vi "FFT1D_LabVIEW.vi"(7 "Iteration":i32, 11 "Samples":i32) -> (3 "Results(s)":dbl format="%.8f")   [LabVIEW 2020]
uses:
  <vilib>/Analysis/NI_AALBase.lvlib
  <vilib>/Analysis/NI_AALPro.lvlib
  ec656ee5-c5d1-4756-bc0c-4372cb75bedf.vi
  88f9a4a6-1eb4-4671-a21a-3a41d51d2300.vi
  <vilib>/Analysis/2dsp.llb/Complex FFT.vi
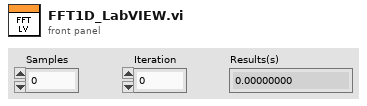
[diagram p1: front panel]
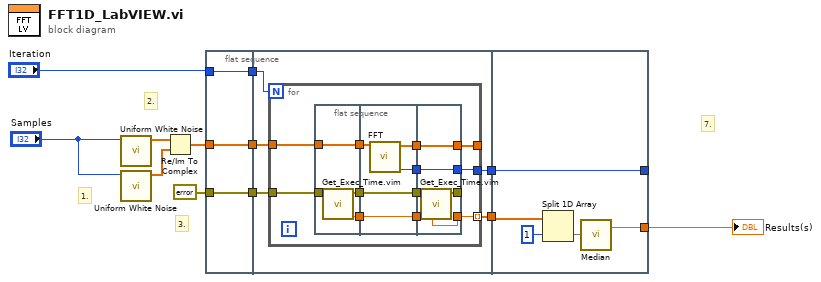
[diagram p0: block diagram]
diagram:
  # "3."
  # "7."
  # "2."
  # "1."
  n1 = call <vilib>:"Uniform White Noise.vi"("samples"="Samples") -> ("uniform white noise"=w2:dbl[])  [unwired: 9 in, 1 out]
  n2 = call <vilib>:"Uniform White Noise.vi"("samples"="Samples") -> ("uniform white noise"=w3:dbl[])  [unwired: 9 in, 1 out]
  n3 = Re/Im To Complex(1:w3, 2:w2) -> (0:w5:cdb[])
  n4 = flat-sequence {
    tunnel: errorcluster {"status"=FALSE, "code"=0, "source"=""} ("error out") -> [w13]
    tunnel: w5 -> [w14]
    tunnel: "Iteration" -> [w15]
    tunnel: [w15] -> w11
    tunnel: [w14] -> w10
    tunnel: [w13] -> w9
    tunnel: [w18] -> w8
    tunnel: w11 -> [w17]
    tunnel: w10 -> [w20]
    tunnel: w9 -> [w19]
    tunnel: [w16] -> w7
    tunnel: [w52] -> _
    tunnel: w8 -> [w52]
    tunnel: [w48] -> w6
    tunnel: w7 -> [w51]
    frame #0 {
    }
    frame #1 {
      n5 = for {
        N: w17 -> [_]
        tunnel: w20 -> [w31]
        tunnel: w19 -> [w29]
        tunnel: [w32] -> w18
        tunnel: [w30] -> _
        tunnel: [w21] -> w16 mode=indexing
        n6 = flat-sequence {
          tunnel: w29 -> [w35]
          tunnel: w31 -> [w36]
          tunnel: [w36] -> w28
          tunnel: [w34] -> w27
          tunnel: [w33] -> w22
          tunnel: w28 -> [w40]
          tunnel: w27 -> [w38]
          tunnel: [w41] -> w26
          tunnel: [w39] -> w25
          tunnel: [w38] -> w24
          tunnel: [w37] -> w23
          tunnel: w22 -> [w37]
          tunnel: [w44] -> _
          tunnel: [w46] -> w30
          tunnel: [w47] -> w32
          tunnel: w26 -> [w47]
          tunnel: w25 -> [w46]
          tunnel: w24 -> [w45]
          tunnel: w23 -> [w43]
          tunnel: [w42] -> w21
          frame #0 {
            n7 = call "Get_Exec_Time.vim"("error in (no error)"=w35) -> ("T(n)"=w33:dbl, "error out"=w34:errorcluster)  [unwired: 6 in, 1 out]
          }
          frame #1 {
            n8 = call-poly <vilib>:"FFT.vi"("X"=w40) -> ("error"=w41:i32, "FFT {X}"=w39:cdb[])  [unwired: 9 in]
          }
          frame #2 {
            n9 = call "Get_Exec_Time.vim"("T(n-1)"=w43, "error in (no error)"=w45) -> ("error out"=w44:errorcluster, "dT"=w42:dbl)  [unwired: 5 in, 1 out]
          }
        }
      }
    }
    frame #2 {
      n10 = Split 1D Array(array=w51, index=1) -> (second subarray=w49:dbl[])  [unwired: 1 out]
      n11 = call <vilib>:"Median.vi"("X"=w49) -> ("median"=w48:dbl)  [unwired: 1 out]
    }
  }
  "Results(s)" <- w6
